vi "Convert Filter IDs String to Array.vi"(11 "Filter IDs":string caption="Filter IDs (format = x<ID>, comma seperated, ID x0 = Bus Error)") -> (3 "Filter IDs":u32[](array[numeric]))   [LabVIEW 2019, in "CAN Stream Support Workspace Shared.lvlib"]
uses:
  CAN Stream Support Workspace Shared.lvlib
  <vilib>/Utility/error.llb/Trim Whitespace One-Sided.vi
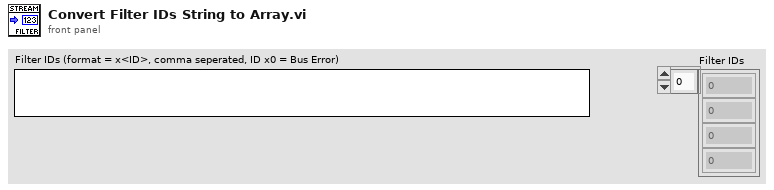
[diagram p1: front panel]
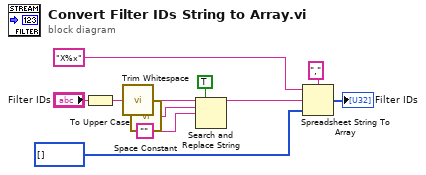
[diagram p0: block diagram]
diagram:
  n1 = To Upper Case(1:"Filter IDs") -> (0:w8:string)
  n2 = call <vilib>:"Trim Whitespace.vi"("string"=w8) -> ("trimmed string"=w5:string)  [unwired: 1 in]
  n3 = call <vilib>:"Space Constant.vi"() -> ("String"=w2:string)
  n4 = Search and Replace String(replace all?=TRUE ("replace all? (F)"), input string=w5, search string=w2, replace string="") -> (result string=w4:string)  [unwired: 4 in, 3 out]
  n5 = Spreadsheet String To Array(delimiter (Tab)=",", format string="X%x", spreadsheet string=w4, array type (2D Dbl)=u32[] []) -> (array=→"Filter IDs":u32[])
